vi "csv数据转JOSN发送.vi"() -> ()   [LabVIEW 2016]
uses:
  <vilib>/httpClient/POSTBuffer.vi
  <vilib>/Utility/file.llb/Read Delimited Spreadsheet (DBL).vi
  <vilib>/httpClient/LabVIEWHTTPClient.lvlib
  <vilib>/Utility/config.llb/NI_LVConfig.lvlib
panel:
  out "队列中元素数量":i32
  in  "开机启动":bool
  in  "拆分间隔(默认100)":i32=100
  out "data":T1={"equipmentCode"="AH CODCR", "packageCount"=0, "packageNum"=0, "time"="2021-05-08 14-02-02", "data"=[]}
  out "body":string caption="体部"
  out "headers":string caption="头部"
  in  "url":string="127.0.0.1:1000"
  out "error out":errorcluster
  in  "equipmentCode":string="AH CODCR"
  in  "time":string="2021-05-08 14:02:02"
  in  "查询":bool
  in  "data path":path=path "C:/Users/TinkPad/Desktop/光谱数据"
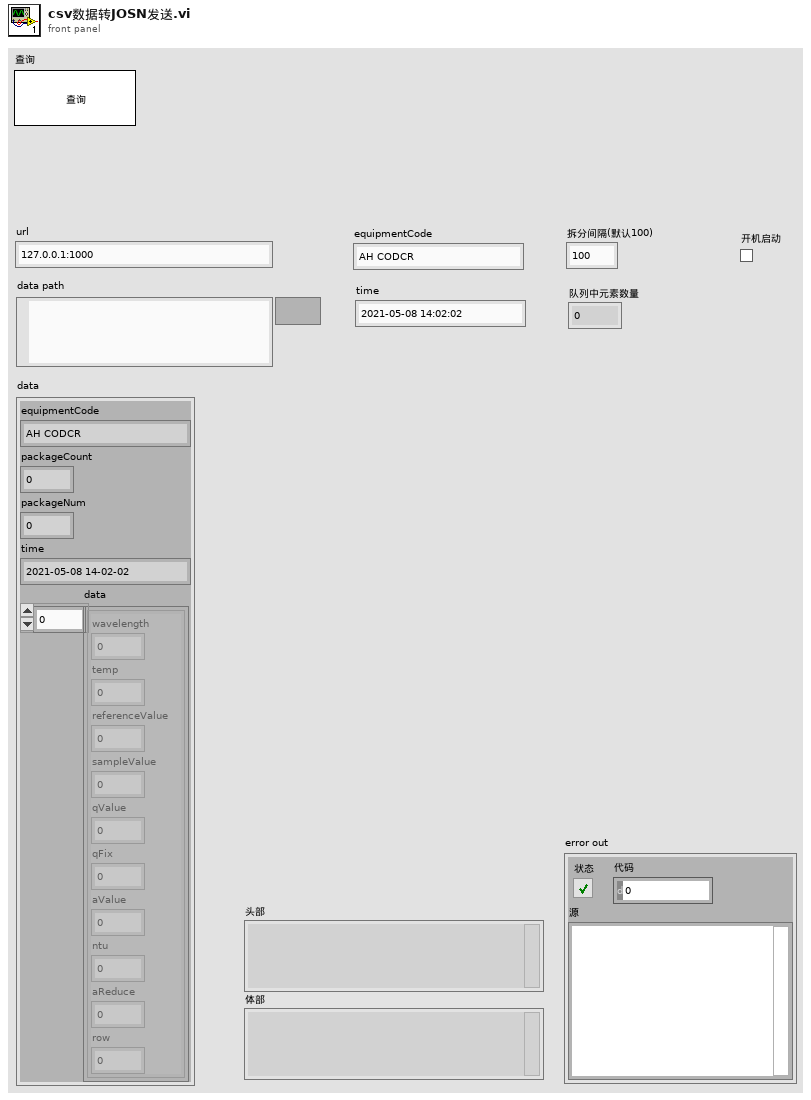
[diagram p1: front panel]
types:
  T1 = cluster{"equipmentCode":string, "packageCount":u32, "packageNum":u32, "time":string, "data":cluster{"wavelength":ext, "temp":ext, "referenceValue":ext, "sampleValue":ext, "qValue":ext, "qFix":ext, "aValue":ext, "ntu":ext, "aReduce":ext, "row":u32}[]}
  T2 = typedef "NI_LVConfig.lvlib/Config Data RefNum.ctl" = refnum<k1>
  T3 = cluster{"wavelength":dbl, "temp":dbl, "referenceValue":dbl, "sampleValue":dbl, "qValue":dbl, "qFix":dbl, "aValue":dbl, "ntu":dbl, "aReduce":dbl, "row":dbl}
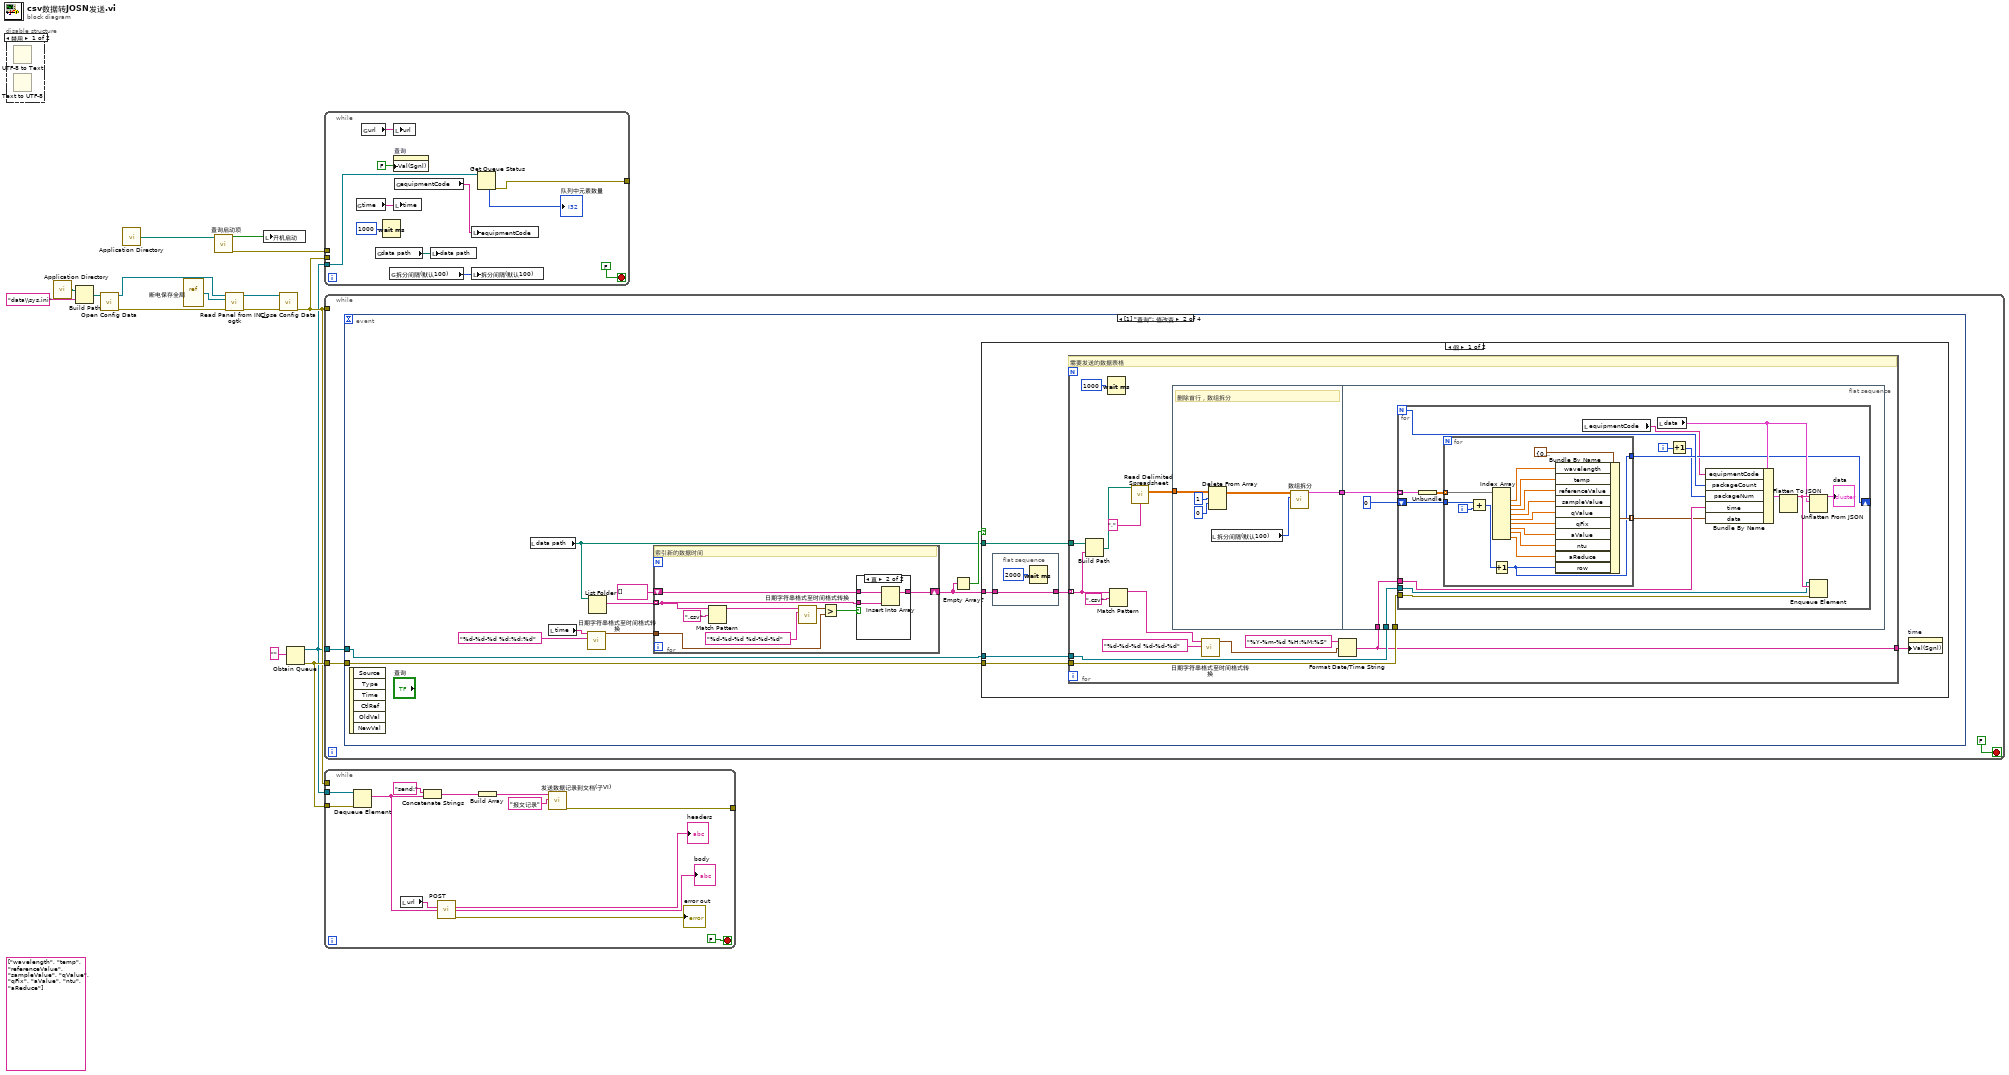
[diagram p0: block diagram]
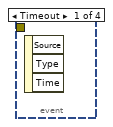
[diagram p3: hidden frame]
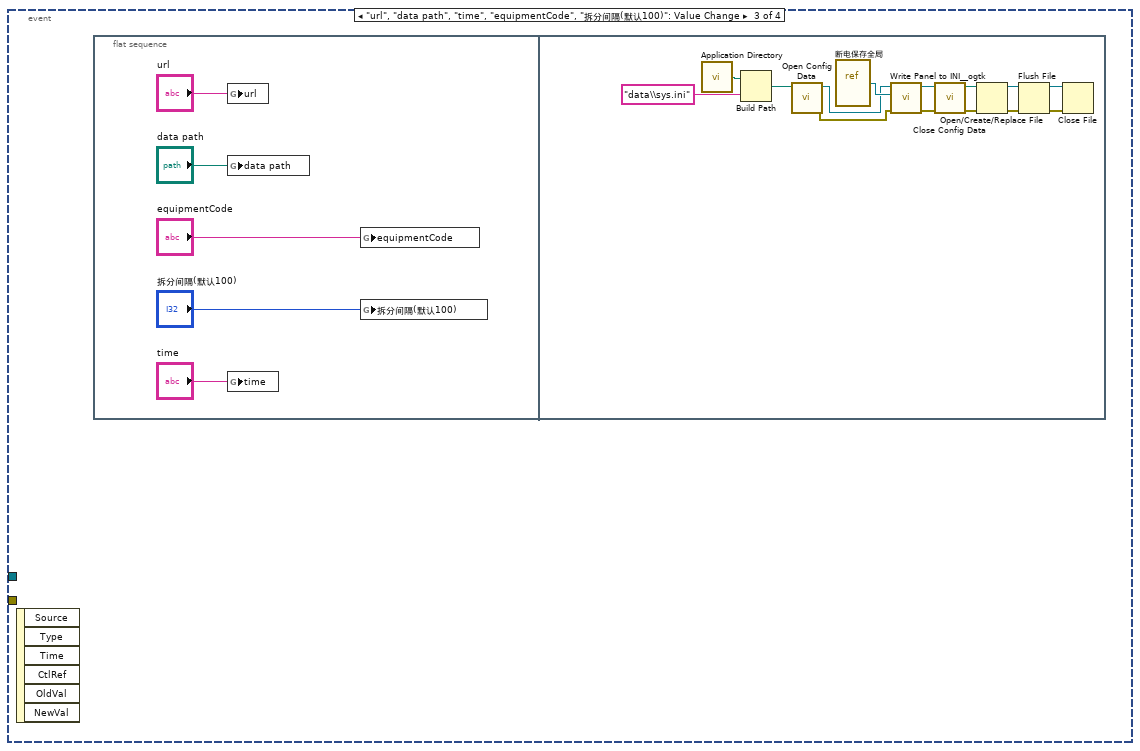
[diagram p6: hidden frame]
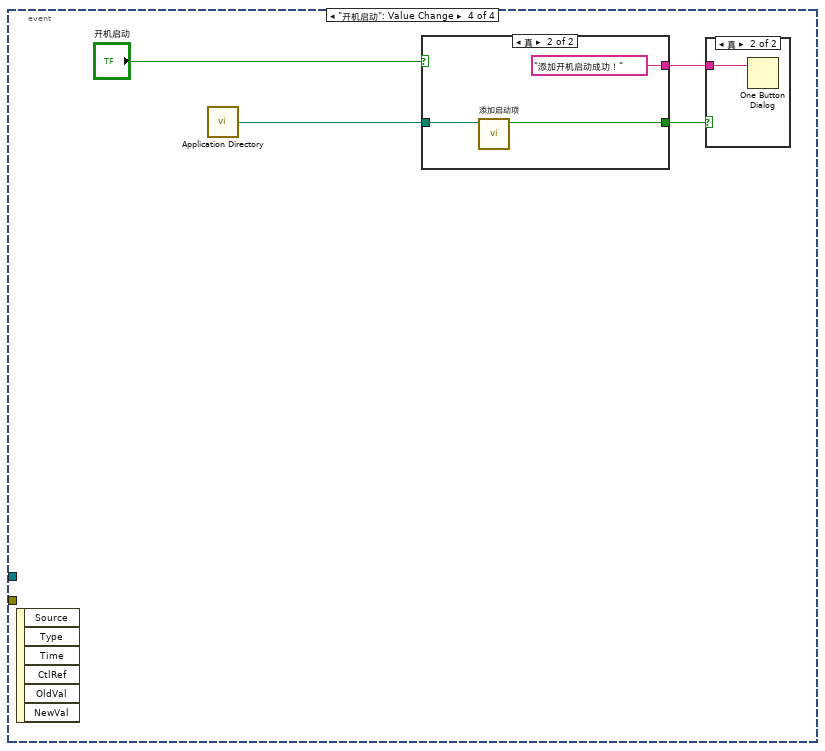
[diagram p7: hidden frame]
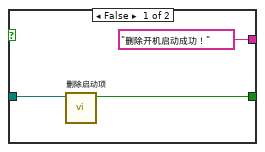
[diagram p9: hidden frame]
diagram:
  (unwired) string[] ["wavelength", "temp", "referenceValue", "sampleValue", "qValue", "qFix", "aValue", "ntu", "aReduce"] ("新元素/子数组")
  n1 = disable-structure shown="禁用" {
    frame Disabled {
      n2 = UTF-8 to Text() -> ()  [unwired: 3 in, 2 out]
      n3 = Text to UTF-8() -> ()  [unwired: 3 in, 2 out]
    }
    frame Enabled {
    }
  }
  n4 = call <vilib>:"Application Directory.vi"() -> ("Application Directory"=w10:path)
  n5 = Build Path(base path=w10, name or relative path="data\\sys.ini" ("名称或相对路径")) -> (appended path=w9:path)
  n6 = call <vilib>:"Open Config Data.vi"("configuration file path"=w9) -> ("error out"=w13:errorcluster, "refnum"=w12:T2)  [unwired: 8 in, 1 out]
  n7 = call <vilib>:"Application Directory.vi"() -> ("Application Directory"=w3:path)
  n8 = vi-ref "断电保存全局.vi"() -> (w7:refnum<vi>)
  n9 = call "查询启动项.vi"("启动文件路径"=w3) -> ("error out"=w2:errorcluster, "包含启动项"=w4:bool)  [unwired: 9 in]
  n10 = call <userlib>:"Read Panel from INI__ogtk.vi"("error in (no error)"=w13, "VI ref"=w7, "refnum"=w12) -> ("error out"=w8:errorcluster, "refnum out"=w11:T2)  [unwired: 7 in]
  n11 = local write "开机启动"(w4) -> ()
  n12 = call <vilib>:"Close Config Data.vi"("error in (no error)"=w8, "refnum"=w11) -> ("error out"=w5:errorcluster)  [unwired: 8 in, 1 out]
  n13 = Obtain Queue(element data type="") -> (queue out=w1:refnum<queue>, error out=w15:errorcluster)  [unwired: 4 in, 1 out]
  n14 = while {
    tunnel: w5 -> [_]
    tunnel: w2 -> [_]
    tunnel: w1 -> [w18]
    tunnel: [w16] -> _
    stop <- FALSE stop-if-true
    n15 = global read "断电保存全局.vi" "time"() -> (w22:string)
    n16 = global read "断电保存全局.vi" "url"() -> (w24:string)
    n17 = global read "断电保存全局.vi" "data path"() -> (w23:path)
    n18 = Wait (ms)(milliseconds to wait=u32 1000 ("等待时间（毫秒）")) -> ()  [unwired: 1 out]
    n19 = global read "断电保存全局.vi" "拆分间隔(默认100)"() -> (w20:i32)
    n20 = local write "url"(w24) -> ()
    n21 = property on="查询" class="Bool (严格)"("Val(Sgnl)"=FALSE ("值(信号)")) -> ()  [unwired: 2 in, 2 out]
    n22 = local write "time"(w22) -> ()
    n23 = global read "断电保存全局.vi" "equipmentCode"() -> (w21:string)
    n24 = local write "data path"(w23) -> ()
    n25 = local write "equipmentCode"(w21) -> ()
    n26 = local write "拆分间隔(默认100)"(w20) -> ()
    n27 = Get Queue Status(queue=w18) -> (error out=w16:errorcluster, # elements in queue=→"队列中元素数量":i32)  [unwired: 2 in, 6 out]
  }
  n28 = while {
    tunnel: w1 -> [w29]
    tunnel: w15 -> [w28]
    tunnel: w5 -> [_]
    stop <- FALSE stop-if-true
    n29 = event shown="[1] \"查询\": 值改变" {
      selector: _ -> [_ _ _ _]
      dyn-events: _ -> [_ _ _ _]
      timeout: _ -> [_ _ _ _]
      tunnel: w29 -> [_ w34 _ _]
      tunnel: w28 -> [_ w33 _ _]
      event Timeout {
        n30 = event-data() -> ()  [unwired: 1 in, 3 out]
      }
      event "查询": Value Change {
        n31 = event-data() -> ()  [unwired: 1 in, 6 out]
        n32 = local read "data path"() -> (w31:path)
        n33 = local read "time"() -> (w30:string)
        n34 = call "日期字符串格式至时间格式转换.vi"("格式字符串"="%d-%d-%d %d:%d:%d", "time"=w30) -> ("time stamp"=w37:timestamp)  [unwired: 9 in]
        n35 = List Folder(path=w31) -> (filenames=w39:string[])  [unwired: 3 in, 3 out]
        n36 = for {
          tunnel: w39 -> [w111] mode=indexing
          tunnel: w37 -> [w113]
          shift-right: [w109] -> w36
          shift-left: string[] [] ("文件名") -> [w110]
          # "索引新的数据时间"
          n37 = Match Pattern(string=w111, regular expression=".csv" ("正则表达式")) -> (before substring=w108:string)  [unwired: 1 in, 3 out]
          n38 = call "日期字符串格式至时间格式转换.vi"("格式字符串"="%d-%d-%d %d-%d-%d", "time"=w108) -> ("time stamp"=w107:timestamp)  [unwired: 9 in]
          n39 = Greater?(x=w107, y=w113) -> (0:w112:bool)
          n40 = case shown="真" w112 {
            tunnel: w111 -> [_ w117]
            tunnel: w110 -> [w115 w118]
            tunnel: [w115 w116] -> w109
            frame False {
            }
            frame True {
              n41 = Insert Into Array(array=w118, new element=w117) -> (w116:string[])  [unwired: 1 in]
            }
          }
        }
        n42 = Empty Array?(array=w36) -> (empty?=w35:bool)
        n43 = case shown="假" w35 {
          tunnel: w31 -> [w43 _]
          tunnel: w36 -> [w42 _]
          tunnel: w34 -> [w45 _]
          tunnel: w33 -> [w44 _]
          frame False {
            n44 = flat-sequence {
              tunnel: w42 -> [w46]
              tunnel: [w46] -> w41
              frame #0 {
                n45 = Wait (ms)(milliseconds to wait=u32 2000 ("等待时间（毫秒）")) -> ()  [unwired: 1 out]
              }
            }
            n46 = for {
              tunnel: w43 -> [w62]
              tunnel: w41 -> [w61] mode=indexing
              tunnel: w45 -> [w59]
              tunnel: w44 -> [w58]
              tunnel: [w48] -> w40
              # "需要发送的数据表格"
              n47 = Build Path(base path=w62, name or relative path=w61) -> (appended path=w52:path)
              n48 = Wait (ms)(milliseconds to wait=u32 1000 ("等待时间（毫秒）")) -> ()  [unwired: 1 out]
              n49 = Match Pattern(string=w61, regular expression=".csv" ("正则表达式")) -> (before substring=w56:string)  [unwired: 1 in, 3 out]
              n50 = call-poly <vilib>:"Read Delimited Spreadsheet.vi"("file path (dialog if empty)"=w52, "delimiter (\\t)"="," ("delimiter (\\t)")) -> ("all rows"=w51:dbl[][])  [unwired: 8 in, 5 out]
              n51 = flat-sequence {
                tunnel: w51 -> [w68]
                tunnel: [w64] -> w49
                tunnel: w59 -> [w73]
                tunnel: w58 -> [w72]
                tunnel: w48 -> [w71]
                tunnel: w49 -> [w69]
                frame #0 {
                  # "删除首行，数组拆分"
                  n52 = Delete From Array(array=w68, length=1 ("长度"), index (row)=0 ("索引 (行)")) -> (array with subset deleted=w65:dbl[][])  [unwired: 1 in, 1 out]
                  n53 = local read "拆分间隔(默认100)"() -> (w63:i32)
                  n54 = call "数组拆分.vi"("拆分间隔"=w63, "all rows"=w65) -> ("数组"=w64:cluster{dbl[][]}[])  [unwired: 9 in]
                }
                frame #1 {
                  n55 = for {
                    N -> [w82]
                    tunnel: w69 -> [w76] mode=indexing
                    tunnel: w73 -> [w85]
                    tunnel: w72 -> [w84]
                    tunnel: w71 -> [w83]
                    shift-right: [w79] -> _
                    shift-left: 0 -> [w80]
                    i -> [w78]
                    n56 = Unbundle(w76) -> (w75:dbl[][])
                    n57 = for {
                      tunnel: w75 -> [w104] mode=indexing
                      tunnel: [w94] -> w81 mode=indexing
                      tunnel: w80 -> [w93]
                      tunnel: [w90] -> w79
                      i -> [w92]
                      n58 = Add(x=w93, y=w92) -> (x+y=w91:i32)
                      n59 = Index Array(array=w104) -> (element #1=w103:dbl, element #2=w102:dbl, element #3=w101:dbl, element #4=w100:dbl, element #5=w99:dbl, element #6=w98:dbl, element #7=w97:dbl, element #8=w96:dbl, element #9=w95:dbl)  [unwired: 9 in]
                      n60 = Increment(x=w91) -> (x+1=w90:i32)
                      n61 = Bundle By Name(cluster=T3 {"wavelength"=0.0, "temp"=0.0, "referenceValue"=0.0, "sampleValue"=0.0, "qValue"=0.0, "qFix"=0.0, "aValue"=0.0, "ntu"=0.0, "aReduce"=0.0, "row"=0.0} ("data"), "wavelength"=w103, "temp"=w102, "referenceValue"=w101, "sampleValue"=w100, "qValue"=w99, "qFix"=w98, "aValue"=w97, "ntu"=w96, "aReduce"=w95, "row"=w90) -> (w94:T3)
                    }
                    n62 = local read "equipmentCode"() -> (w74:string)
                    n63 = local read "data"() -> (w87:T1)
                    n64 = Increment(x=w78) -> (x+1=w77:i32)
                    n65 = Bundle By Name(cluster=w87, "equipmentCode"=w74, "packageCount"=w82, "packageNum"=w77, "time"=w83, "data"=w81) -> (w89:T1)
                    n66 = Flatten To JSON(anything=w89) -> (JSON string=w88:string)  [unwired: 2 in, 1 out]
                    n67 = Unflatten From JSON(JSON string=w88, type and defaults=w87) -> (value=→"data":T1)  [unwired: 5 in, 1 out]
                    n68 = Enqueue Element(queue=w85, element=w88, error in (no error)=w84) -> ()  [unwired: 1 in, 3 out]
                  }
                }
              }
              n69 = call "日期字符串格式至时间格式转换.vi"("格式字符串"="%d-%d-%d %d-%d-%d", "time"=w56) -> ("time stamp"=w53:timestamp)  [unwired: 9 in]
              n70 = Format Date/Time String(time format string (%c)="%Y-%m-%d %H:%M:%S" ("时间格式字符串(%c)"), seconds (now)=w53) -> (date/time string=w48:string)  [unwired: 1 in]
            }
            n71 = property on="time" class="Str"("Val(Sgnl)"=w40) -> ()  [unwired: 2 in, 2 out]
          }
          frame True {
          }
        }
      }
      event "url", "data path", "time", "equipmentCode", "拆分间隔(默认100)": Value Change {
        n72 = event-data() -> ()  [unwired: 1 in, 6 out]
        n73 = flat-sequence {
          frame #0 {
            n74 = global write "断电保存全局.vi" "url"("url") -> ()
            n75 = global write "断电保存全局.vi" "data path"("data path") -> ()
            n76 = global write "断电保存全局.vi" "time"("time") -> ()
            n77 = global write "断电保存全局.vi" "equipmentCode"("equipmentCode") -> ()
            n78 = global write "断电保存全局.vi" "拆分间隔(默认100)"("拆分间隔(默认100)") -> ()
          }
          frame #1 {
            n79 = call <vilib>:"Application Directory.vi"() -> ("Application Directory"=w124:path)
            n80 = Build Path(base path=w124, name or relative path="data\\sys.ini" ("名称或相对路径")) -> (appended path=w126:path)
            n81 = call <vilib>:"Open Config Data.vi"("configuration file path"=w126) -> ("error out"=w130:errorcluster, "refnum"=w127:T2)  [unwired: 8 in, 1 out]
            n82 = vi-ref "断电保存全局.vi"() -> (w128:refnum<vi>)
            n83 = call <userlib>:"Write Panel to INI__ogtk.vi"("error in (no error)"=w130, "VI ref"=w128, "refnum"=w127) -> ("error out"=w131:errorcluster, "refnum out"=w129:T2)  [unwired: 7 in]
            n84 = call <vilib>:"Close Config Data.vi"("error in (no error)"=w131, "refnum"=w129) -> ("error out"=w136:errorcluster, "file path"=w137:path)  [unwired: 8 in]
            n85 = Open/Create/Replace File(file path (use dialog)=w137, error in=w136) -> (refnum out=w133:refnum<file>, error out=w132:errorcluster)  [unwired: 4 in, 1 out]
            n86 = Flush File(refnum=w133, error in=w132) -> (refnum out=w134:refnum<file>, error out=w135:errorcluster)
            n87 = Close File(refnum=w134, error in=w135) -> ()  [unwired: 2 out]
          }
        }
      }
      event "开机启动": Value Change {
        n88 = event-data() -> ()  [unwired: 1 in, 6 out]
        n89 = call <vilib>:"Application Directory.vi"() -> ("Application Directory"=w140:path)
        n90 = case shown="真" "开机启动" {
          tunnel: w140 -> [w145 w148]
          tunnel: [w144 w147] -> w139
          tunnel: ["删除开机启动成功！" ("消息") "添加开机启动成功！" ("消息")] -> w138
          frame False {
            n91 = call "删除启动项.vi"("启动文件路径"=w145) -> ("删除标记"=w144:bool)  [unwired: 9 in, 1 out]
          }
          frame True {
            n92 = call "添加启动项.vi"("启动文件路径"=w148) -> ("添加成功标记"=w147:bool)  [unwired: 9 in, 1 out]
          }
        }
        n93 = case shown="真" w139 {
          tunnel: w138 -> [_ w142]
          frame False {
          }
          frame True {
            n94 = One Button Dialog(message=w142) -> ()  [unwired: 1 in, 1 out]
          }
        }
      }
    }
  }
  n95 = while {
    tunnel: w1 -> [w150]
    tunnel: w15 -> [w149]
    tunnel: w5 -> [_]
    tunnel: [w151] -> _
    stop <- FALSE stop-if-true
    n96 = Dequeue Element(queue=w150, error in (no error)=w149) -> (element=w154:string)  [unwired: 1 in, 3 out]
    n97 = local read "url"() -> (w157:string)
    n98 = Concatenate Strings("send:" ("字符串"), w154) -> (w155:string)
    n99 = call-poly <vilib>:"POST.vi"("url"=w157, "buffer"=w154) -> ("headers"=→"headers":string, "body"=→"body":string, "error out"=→"error out":errorcluster)  [unwired: 10 in, 1 out]
    n100 = Build Array(w155) -> (w153:string[])
    n101 = call "发送数据记录到文档(子VI).vi"("字符串"="报文记录", "数组"=w153) -> ("错误输出"=w151:errorcluster)  [unwired: 8 in]
  }
